vi "FRIC_navX_Get_BoardInformation.vi"(5 "Device Number":T1, 7 "Update":bool) -> (2 "Board Information":T4 {"Board"."Hardware Revision" items=["navX-MXP"=33, "navX-Micro"=40]; "Omnimount Config" items=["DEFAULT", "X_UP", "X_DOWN", "Y_UP", "Y_DOWN", "Z_UP", "Z_DOWN"]})   [LabVIEW 2015]
doc: "This navX VI will return the current Board Information.\nWho Am I\nHardware Revision\nFirmware Major and Minor\nCapability\nOmnimount Config"
uses:
  _TypeDefs/Flags/Z900_navX_Flags_HardwareRevTypeDef.ctl
  _TypeDefs/Flags/Z900_navX_Flags_OmnimountConfigTypeDef.ctl
  _TypeDefs/FRIC_navX_DeviceNumbersTypeDef.ctl
  _TypeDefs/Z900_navX_DeviceRegisters.ctl
  _TypeDefs/Flags/Z900_navX_Flags_CapabilityTypeDef.ctl
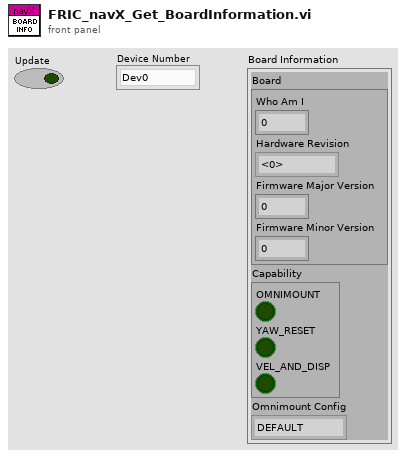
[diagram p1: front panel]
types:
  T1 = typedef "FRIC_navX_DeviceNumbersTypeDef.ctl" = enum16{"Dev0", "Dev1", "Dev2", "Dev3", "Dev4", "Dev5", "Dev6", "Dev7", "Dev8", "Dev9", "Dev10"}
  T2 = typedef "Z900_navX_Flags_HardwareRevTypeDef.ctl" = u8
  T3 = typedef "Z900_navX_Flags_OmnimountConfigTypeDef.ctl" = u8
  T4 = cluster{"Board":cluster{"Who Am I":u8, "Hardware Revision":T2, "Firmware Major Version":u8, "Firmware Minor Version":u8}, "Capability":cluster{"OMNIMOUNT":bool, "YAW_RESET":bool, "VEL_AND_DISP":bool}, "Omnimount Config":T3}
  T5 = cluster{"Who Am I":u8, "Hardware Revision":T2, "Firmware Major Version":u8, "Firmware Minor Version":u8}
  T6 = cluster{"OMNIMOUNT":bool, "YAW_RESET":bool, "VEL_AND_DISP":bool}
  T7 = typedef "Z900_navX_DeviceRegisters.ctl" = u8
  T8 = typedef "Z900_navX_Flags_CapabilityTypeDef.ctl" = u16
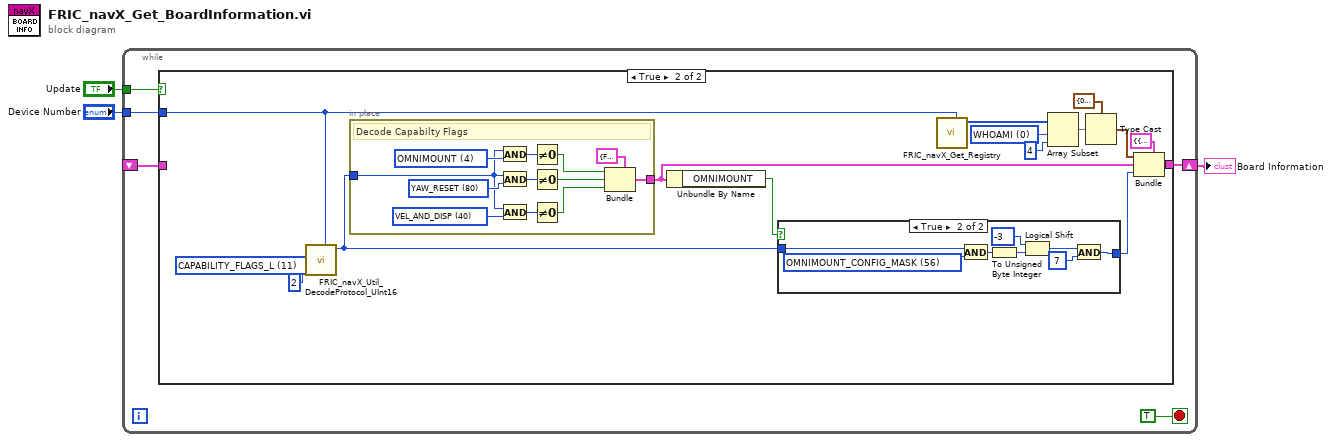
[diagram p0: block diagram]
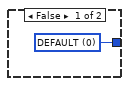
[diagram p3: hidden frame]
diagram:
  n1 = while {
    shift-right: [w8] -> w2
    shift-left: _ -> [w7]
    tunnel: "Update" -> [w6]
    tunnel: "Device Number" -> [w4]
    stop <- TRUE stop-if-true
    n2 = case shown="True" w6 {
      tunnel: [w9 w11] -> w8
      tunnel: w7 -> [w9 _]
      tunnel: w4 -> [_ w10]
      frame False {
      }
      frame True {
        w12 = T7 0 items=["WHOAMI"=0, "HW_REV"=1, "FW_VER_MAJOR"=2, "FW_VER_MINOR"=3, "UPDATE_RATE_HZ"=4, "ACCEL_FSR_G"=5, "GYRO_FSR_DPS"=6, "OP_STATUS"=8, "CAL_STATUS"=9, "SELFTEST_STATUS"=10, "CAPABILITY_FLAGS_L"=11, "CAPABILITY_FLAGS_H"=12, "SENSOR_STATUS"=16, "TIMESTAMP"=18, "YAW"=22, "ROLL"=24, "PITCH"=26, "HEADING"=28, "FUSED_HEADING"=30, "ALTITUDE_I"=32, "ALTITUDE_D"=34, "LINERA_ACC_X"=36, "LINERA_ACC_Y"=38, "LINERA_ACC_Z"=40, "QUAT_W"=42, "QUAT_X"=44, "QUAT_Y"=46, "QUAT_Z"=48, "MPU_TEMP_C"=50, "GYRO_X"=52, "GYRO_Y"=54, "GYRO_Z"=56, "ACC_X"=58, "ACC_Y"=60, "ACC_Z"=62, "MAG_X"=64, "MAG_Y"=66, "MAG_Z"=68, "PRESSURE_I"=70, "PRESSURE_D"=72, "PRESSURE_TEMP"=74, "YAW_OFFSET"=76, "QUAT_OFFSET_W"=78, "QUAT_OFFSET_X"=80, "QUAT_OFFSET_Y"=82, "QUAT_OFFSET_Z"=84, "INTEGRATION_CONTROL"=86, "VELOCITY_X"=88, "VELOCITY_Y"=92, "VELOCITY_Z"=96, "DISPLACMENT_X"=100, "DISPLACMENT_Y"=104, "DISPLACEMENT_Z"=108] ("Device Register")
        w16 = T7 11 items=["WHOAMI"=0, "HW_REV"=1, "FW_VER_MAJOR"=2, "FW_VER_MINOR"=3, "UPDATE_RATE_HZ"=4, "ACCEL_FSR_G"=5, "GYRO_FSR_DPS"=6, "OP_STATUS"=8, "CAL_STATUS"=9, "SELFTEST_STATUS"=10, "CAPABILITY_FLAGS_L"=11, "CAPABILITY_FLAGS_H"=12, "SENSOR_STATUS"=16, "TIMESTAMP"=18, "YAW"=22, "ROLL"=24, "PITCH"=26, "HEADING"=28, "FUSED_HEADING"=30, "ALTITUDE_I"=32, "ALTITUDE_D"=34, "LINERA_ACC_X"=36, "LINERA_ACC_Y"=38, "LINERA_ACC_Z"=40, "QUAT_W"=42, "QUAT_X"=44, "QUAT_Y"=46, "QUAT_Z"=48, "MPU_TEMP_C"=50, "GYRO_X"=52, "GYRO_Y"=54, "GYRO_Z"=56, "ACC_X"=58, "ACC_Y"=60, "ACC_Z"=62, "MAG_X"=64, "MAG_Y"=66, "MAG_Z"=68, "PRESSURE_I"=70, "PRESSURE_D"=72, "PRESSURE_TEMP"=74, "YAW_OFFSET"=76, "QUAT_OFFSET_W"=78, "QUAT_OFFSET_X"=80, "QUAT_OFFSET_Y"=82, "QUAT_OFFSET_Z"=84, "INTEGRATION_CONTROL"=86, "VELOCITY_X"=88, "VELOCITY_Y"=92, "VELOCITY_Z"=96, "DISPLACMENT_X"=100, "DISPLACMENT_Y"=104, "DISPLACEMENT_Z"=108] ("Device Register")
        n3 = call "FRIC_navX_Util_DecodeProtocol_UInt16.vi"("Device Number"=w10, "length"=2, "Device Register"=w16) -> ("Value"=w14:u16)  [unwired: 8 in]
        n4 = in-place {
          in-place-border: w14 -> [w36]
          in-place-border: [w34] -> w19
          w39 = T8 40 items=["OMNIMOUNT"=4, "OMNIMOUNT_CONFIG_MASK"=38, "VEL_AND_DISP"=40, "YAW_RESET"=80] ("Capability Flag")
          w40 = T8 80 items=["OMNIMOUNT"=4, "OMNIMOUNT_CONFIG_MASK"=38, "VEL_AND_DISP"=40, "YAW_RESET"=80] ("Capability Flag")
          w45 = T8 4 items=["OMNIMOUNT"=4, "OMNIMOUNT_CONFIG_MASK"=38, "VEL_AND_DISP"=40, "YAW_RESET"=80] ("Capability Flag")
          # "Decode Capabilty Flags"
          n5 = And(x=w36, y=w45) -> (x .and. y?=w44:T8)
          n6 = And(x=w36, y=w40) -> (x .and. y?=w41:T8)
          n7 = And(x=w36, y=w39) -> (x .and. y?=w38:T8)
          n8 = Not Equal To 0?(x=w44) -> (x != 0?=w42:bool)
          n9 = Not Equal To 0?(x=w41) -> (x != 0?=w37:bool)
          n10 = Not Equal To 0?(x=w38) -> (x != 0?=w35:bool)
          n11 = Bundle(cluster=T6 {"OMNIMOUNT"=FALSE, "YAW_RESET"=FALSE, "VEL_AND_DISP"=FALSE}, "OMNIMOUNT"=w42, "YAW_RESET"=w37, "VEL_AND_DISP"=w35) -> (w34:T6)
        }
        n12 = Unbundle By Name(w19) -> ("OMNIMOUNT"=w23:bool)
        n13 = case shown="True" w23 {
          tunnel: [w25 w27] -> w17
          tunnel: w14 -> [_ w33]
          frame False {
            w25 = u8 0 items=["DEFAULT", "X_UP", "X_DOWN", "Y_UP", "Y_DOWN", "Z_UP", "Z_DOWN"] ("OMNIMOUNT_CONFIG")
          }
          frame True {
            w32 = T8 56 items=["OMNIMOUNT"=4, "OMNIMOUNT_CONFIG_MASK"=56, "VEL_AND_DISP"=64, "YAW_RESET"=128] ("Capability Flag")
            n14 = And(x=w33, y=w32) -> (x .and. y?=w31:T8)
            n15 = To Unsigned Byte Integer(number=w31) -> (unsigned 8bit integer=w26:u8)
            n16 = Logical Shift(y=-3, x=w26) -> (x << y=w29:u8)
            n17 = And(x=w29, y=7) -> (x .and. y?=w27:i32)
          }
        }
        n18 = call "FRIC_navX_Get_Registry.vi"("Device Number"=w10) -> ("Registry (out)"=w24:u8[])  [unwired: 9 in, 1 out]
        n19 = Array Subset(array=w24, index=w12, length=4) -> (w22:u8[])
        n20 = Type Cast(type=T5 {"Who Am I"=0, "Hardware Revision"=33, "Firmware Major Version"=0, "Firmware Minor Version"=0}, x=w22) -> (*(type *) &x=w18:T5)
        n21 = Bundle(cluster=T4 {"Board"={"Who Am I"=0, "Hardware Revision"=33, "Firmware Major Version"=0, "Firmware Minor Version"=0}, "Capability"={"OMNIMOUNT"=FALSE, "YAW_RESET"=FALSE, "VEL_AND_DISP"=FALSE}, "Omnimount Config"=0}, "Board"=w18, "Capability"=w19, "Omnimount Config"=w17) -> (w11:T4)
      }
    }
  }
  "Board Information" <- w2
